vi "FPGA_RefCurrSampling.vi"() -> ()   [LabVIEW 2014]
uses:
  <vilib>/rvi/eio/common/nirviEmuTemplateMethod_errors.vi
  <vilib>/rvi/Emulation/niFpgaSctlEmulationGetInTimedLoop.vi
  <vilib>/rvi/Emulation/niFpgaProcessEmulError.vi
  <vilib>/eio/EIONode/EIONode.xnode
panel:
  out "RefCurr":i16
  out "CurrSampleDone?":bool
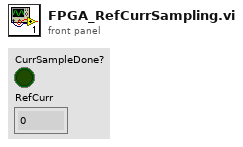
[diagram p1: front panel]
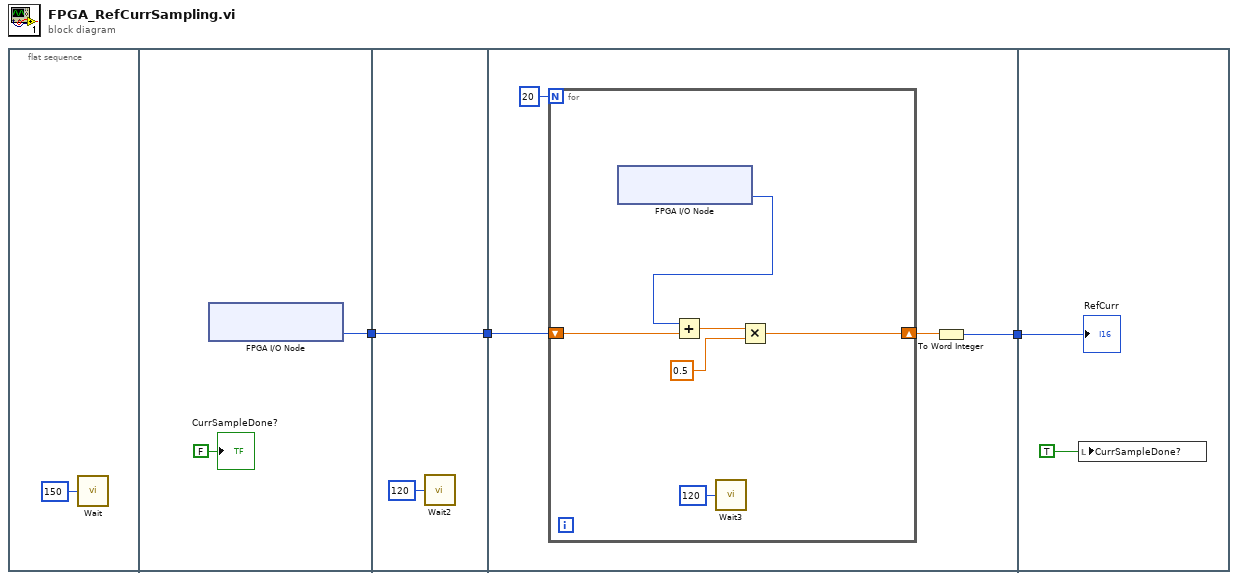
[diagram p0: block diagram]
diagram:
  n1 = flat-sequence {
    tunnel: [w6] -> w3
    tunnel: w3 -> [w8]
    tunnel: [w8] -> w2
    tunnel: w2 -> [w11]
    tunnel: [w9] -> w1
    tunnel: w1 -> [w20]
    frame #0 {
      n2 = call "Wait"("Count(mSec)"=u32 150) -> ()  [unwired: 1 out]
    }
    frame #1 {
      n3 = xnode "FPGA I/O Node"() -> ("Connector0/AI1"=w6:i16)  [unwired: 1 in, 1 out]
      "CurrSampleDone?" <- FALSE
    }
    frame #2 {
      n4 = call "Wait2"("Count(uSec)"=u32 120) -> ()  [unwired: 1 out]
    }
    frame #3 {
      n5 = for {
        N: 20 -> [_]
        shift-right: [w13] -> w10
        shift-left: w11 -> [w17]
        n6 = xnode "FPGA I/O Node"() -> ("Connector0/AI1"=w16:i16)  [unwired: 1 in, 1 out]
        n7 = Add(x=w16, y=w17) -> (x+y=w15:sgl)
        n8 = call "Wait3"("Count(uSec)"=u32 120) -> ()  [unwired: 1 out]
        n9 = Multiply(x=w15, y=sgl 0.5) -> (x*y=w13:sgl)
      }
      n10 = To Word Integer(number=w10) -> (16bit integer=w9:i16)
    }
    frame #4 {
      n11 = local write "CurrSampleDone?"(TRUE) -> ()
      "RefCurr" <- w20
    }
  }
